vi "runSingleScript.vi"(8 "error in (no error)":errorcluster, 10 "runSingleScript":cluster{"Path":path, "HWLoop":bool}, 11 "ExperimentControl in":refnum<class "ExperimentControl.lvclass">) -> (0 "error out":errorcluster, 1 "stopBeforeNext":bool, 2 "stoppedByUser":bool, 3 "ExperimentControl out":refnum<class "ExperimentControl.lvclass">)   [LabVIEW 2009, in "Views.lvlib" / "ExperimentControl.lvlib" / "ExperimentControl.lvclass"]
uses:
  ExperimentControl.lvclass
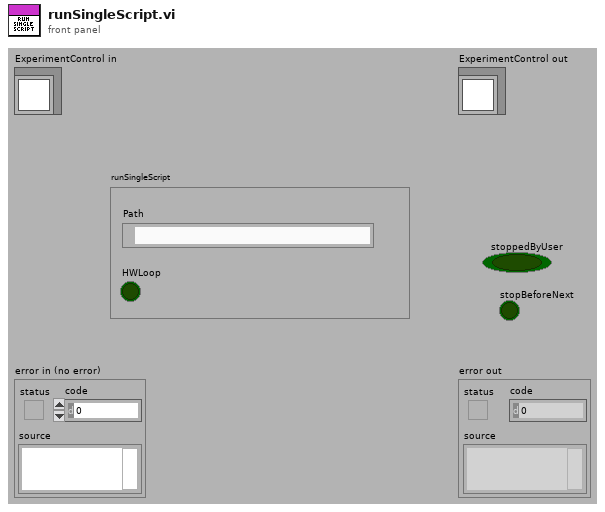
[diagram p1: front panel]
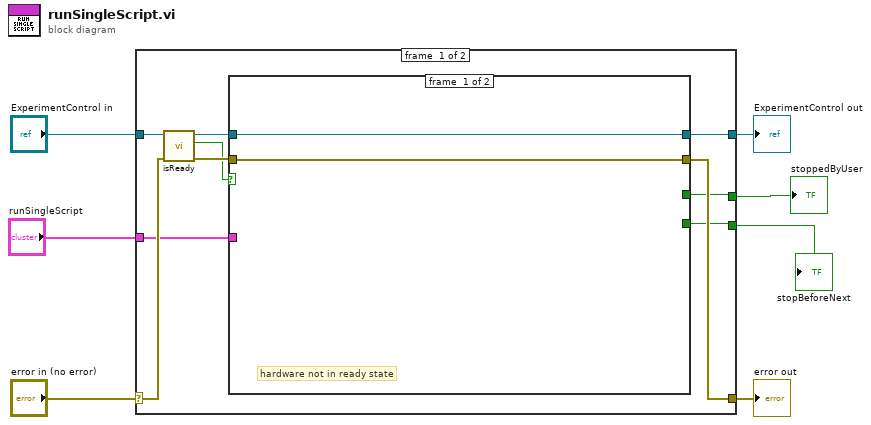
[diagram p0: block diagram]
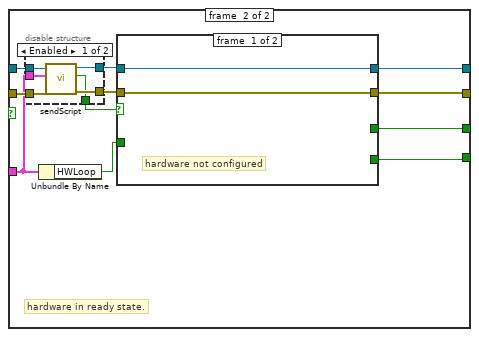
[diagram p2: hidden frame]
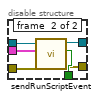
[diagram p3: hidden frame]
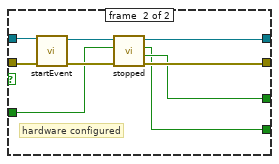
[diagram p4: hidden frame]
diagram:
  n1 = case shown="No Error" "error in (no error)" {
    selector: "error in (no error)" -> [w16 w55]
    tunnel: [w10 w55] -> w6
    tunnel: [w11 w54] -> w4
    tunnel: "ExperimentControl in" -> [w17 w54]
    tunnel: "runSingleScript" -> [w12 _]
    tunnel: [w9 _] -> w2
    tunnel: [w8 _] -> w1
    frame #0 {
      n2 = call "isReady.vi"("error in (no error)"=w16, "ExperimentControl in"=w17) -> ("error out"=w14:errorcluster, "ready?"=w13:bool, "ExperimentControl out"=w15:refnum<class "ExperimentControl.lvclass">)  [unwired: 7 in]
      n3 = case shown="True" w13 {
        tunnel: w15 -> [w19 w25]
        tunnel: w14 -> [w18 w23]
        tunnel: w12 -> [_ w21]
        tunnel: [w19 w30] -> w11
        tunnel: [w18 w29] -> w10
        tunnel: [_ w28] -> w9
        tunnel: [_ w27] -> w8
        frame #0 {
          # "hardware not in ready state"
        }
        frame #1 {
          # "hardware in ready state."
          n4 = disable-structure shown="Enabled" {
            disable-tunnel: w25 -> [w36 w42]
            disable-tunnel: [w35 w37] -> w24
            disable-tunnel: w23 -> [w34 w40]
            disable-tunnel: [w33 w38] -> w22
            disable-tunnel: w21 -> [w32 w41]
            disable-tunnel: [w31 w39] -> w20
            frame #0 {
              n5 = call "sendScript.vi"("error in (no error)"=w34, "runSingleScript"=w32, "ExperimentControl in"=w36) -> ("error out"=w33:errorcluster, "configured"=w31:bool, "ExperimentControl out"=w35:refnum<class "ExperimentControl.lvclass">)  [unwired: 6 in]
            }
            frame #1 {
              n6 = call "sendRunScriptEvent.vi"("error in (no error)"=w40, "runSingleScript"=w41, "ExperimentControl in"=w42) -> ("error out"=w38:errorcluster, "configured"=w39:bool, "ExperimentControl out"=w37:refnum<class "ExperimentControl.lvclass">)  [unwired: 6 in]
            }
          }
          n7 = Unbundle By Name(w21) -> ("HWLoop"=w26:bool)
          n8 = case shown="True" w20 {
            tunnel: w24 -> [w44 w53]
            tunnel: w22 -> [w43 w52]
            tunnel: [w44 w50] -> w30
            tunnel: [w43 w49] -> w29
            tunnel: [_ w47] -> w28
            tunnel: [_ w46] -> w27
            tunnel: w26 -> [_ w45]
            frame #0 {
              # "hardware not configured"
            }
            frame #1 {
              # "hardware configured"
              n9 = call-dynamic "startEvent.vi"("error in (no error)"=w52, "ExperimentControl in"=w53) -> ("error out"=w48:errorcluster, "ExperimentControl out"=w51:refnum<class "ExperimentControl.lvclass">)  [unwired: 8 in]
              n10 = call "stopped.vi"("error in (no error)"=w48, "HWloop"=w45, "ExperimentControl in"=w51) -> ("error out"=w49:errorcluster, "stoppedByUser"=w47:bool, "stopBeforeNext"=w46:bool, "ExperimentControl out"=w50:refnum<class "ExperimentControl.lvclass">)  [unwired: 5 in]
            }
          }
        }
      }
    }
    frame #1 {
    }
  }
  "error out" <- w6
  "ExperimentControl out" <- w4
  "stoppedByUser" <- w2
  "stopBeforeNext" <- w1
